vi "Untitled 1.vi"() -> ()   [LabVIEW 2011]
panel:
  out "x*y":dbl[][](array[numeric])
  out "unsigned 8bit integer":u8[][](array[numeric])
  out "Image 2":T1(plugin-control)
  out "Image":T1(plugin-control)
  in  "transposed array":dbl[][](graph)
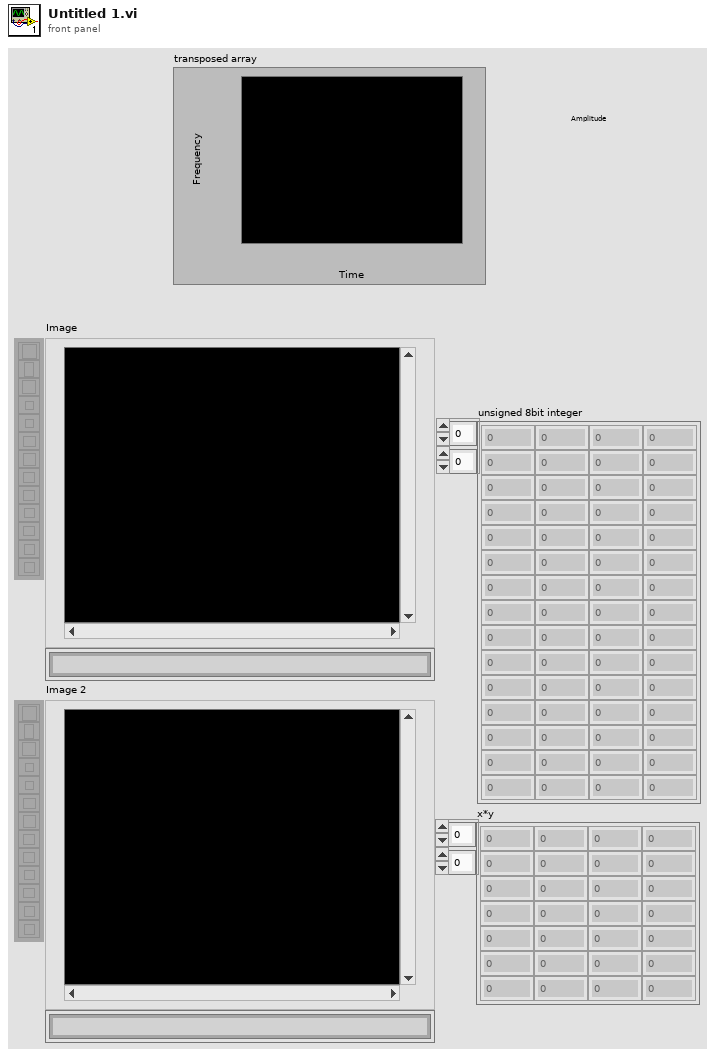
[diagram p1: front panel]
types:
  T1 = typedef "IMAQ Image.ctl" = refnum<image>
  T2 = typedef "Image Type" = u32
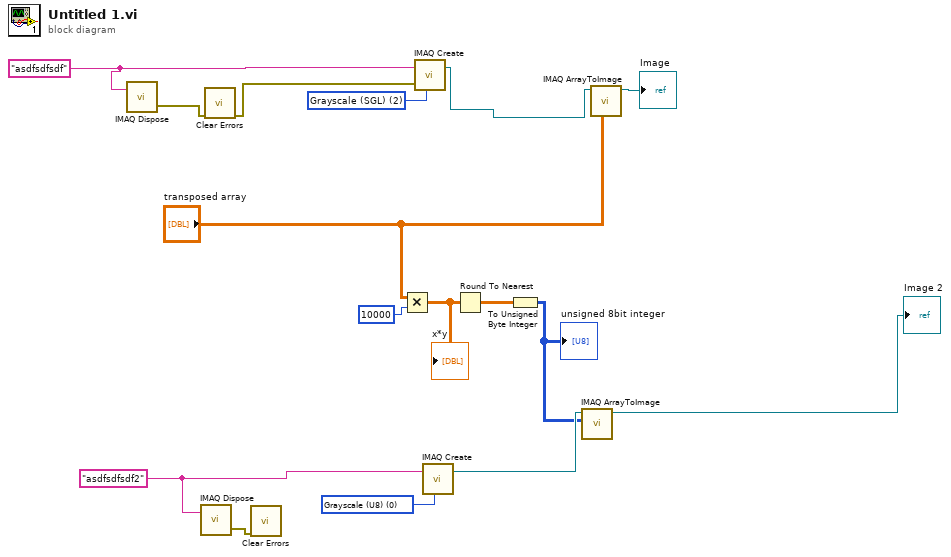
[diagram p0: block diagram]
diagram:
  w14 = T2 0 items=["Grayscale (U8)", "Grayscale (I16)", "Grayscale (SGL)", "Complex (CSG)", "RGB (U32)", "HSL (U32)", "RGB (U64)", "Grayscale (U16)"] ("Image Type")
  w12 = "asdfsdfsdf2" ("Image Name")
  w16 = T2 2 items=["Grayscale (U8)", "Grayscale (I16)", "Grayscale (SGL)", "Complex (CSG)", "RGB (U32)", "HSL (U32)", "RGB (U64)", "Grayscale (U16)"] ("Image Type")
  w13 = "asdfsdfsdf" ("Image Name")
  n1 = call "IMAQ Dispose"("Image"=w13) -> ("error out"=w11:errorcluster)  [unwired: 5 in]
  n2 = call "IMAQ Dispose"("Image"=w12) -> ("error out"=w10:errorcluster)  [unwired: 5 in]
  n3 = call <vilib>:"Clear Errors.vi"("error in (no error)"=w11) -> ("error out"=w8:errorcluster)  [unwired: 6 in]
  n4 = call <vilib>:"Clear Errors.vi"("error in (no error)"=w10) -> ()  [unwired: 6 in, 1 out]
  n5 = Multiply(x="transposed array", y=10000) -> (x*y=w5:dbl[][])
  "x*y" <- w5
  n6 = call "IMAQ Create"("Image Name"=w13, "Image Type"=w16, "error in (no error)"=w8) -> ("New Image"=w15:T1)  [unwired: 2 in, 1 out]
  n7 = call "IMAQ Create"("Image Name"=w12, "Image Type"=w14) -> ("New Image"=w3:T1)  [unwired: 3 in, 1 out]
  n8 = Round To Nearest(number=w5) -> (nearest integer value=w4:dbl[][])
  n9 = To Unsigned Byte Integer(number=w4) -> (unsigned 8bit integer=w1:u8[][])
  "unsigned 8bit integer" <- w1
  n10 = call "IMAQ ArrayToImage"("Image Pixels (U8)"=w1, "Image"=w3) -> ("Image Out"=→"Image 2":T1)  [unwired: 8 in, 1 out]
  n11 = call "IMAQ ArrayToImage"("Image Pixels (Float)"="transposed array", "Image"=w15) -> ("Image Out"=→"Image":T1)  [unwired: 8 in, 1 out]
